vi "XML_FF_writeClassList.vi"(8 "error in (no error)":errorcluster, 10 "ClassList":string[](array[string]), 11 "DOM document in":refnum<k20>) -> (0 "error out":errorcluster, 3 "DOM document out":refnum<k20>)   [LabVIEW 2016, in "XML_EEG_Features.lvlib"]
uses:
  XML_EEG_Features.lvlib
  <vilib>/xml/NI_XML.lvlib
  <resource>/objmgr/DOMUserDefRef.rc
panel:
  # "This VI is a part of BCI Design library, http://www.ru-bci.org \nCopyright © 2020, Sotnikov Peter, All rights reserved. License: CC BY-NC 4.0"
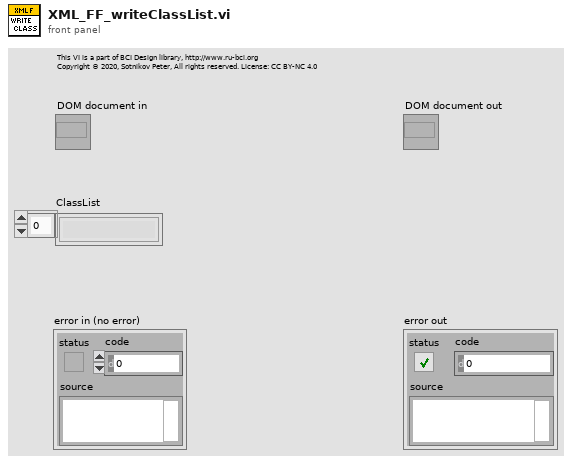
[diagram p1: front panel]
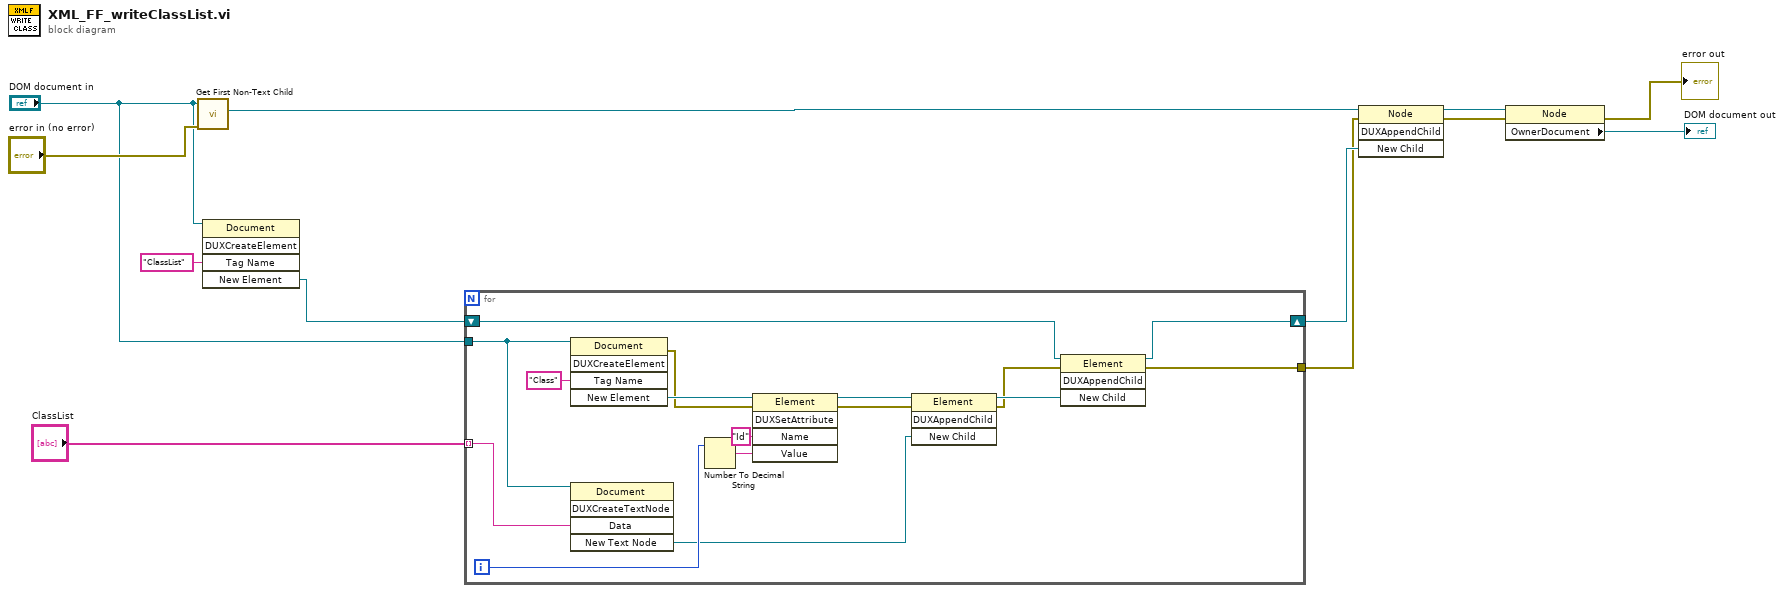
[diagram p0: block diagram]
diagram:
  n1 = call <vilib>:"Get First Non-Text Child.vi"("error in (no error)"="error in (no error)", "node in"="DOM document in") -> ("child node"=w6:refnum<k20>)  [unwired: 6 in, 3 out]
  n2 = invoke class="Document" method="DUXCreateElement"(reference="DOM document in", "Tag Name"="ClassList") -> ("New Element"=w8:refnum<k20>)  [unwired: 3 in, 4 out]
  n3 = for {
    tunnel: "ClassList" -> [w26] mode=indexing
    tunnel: "DOM document in" -> [w27]
    shift-right: [w16] -> w7
    shift-left: w8 -> [w17]
    tunnel: [w13] -> w3
    i -> [w23]
    n4 = invoke class="Document" method="DUXCreateElement"(reference=w27, "Tag Name"="Class") -> (error out=w21:errorcluster, "New Element"=w25:refnum<k20>)  [unwired: 3 in, 3 out]
    n5 = invoke class="Document" method="DUXCreateTextNode"(reference=w27, "Data"=w26) -> ("New Text Node"=w19:refnum<k20>)  [unwired: 3 in, 4 out]
    n6 = Number To Decimal String(number=w23) -> (decimal integer string=w24:string)  [unwired: 1 in]
    n7 = invoke class="Element" method="DUXSetAttribute"(reference=w25, error in=w21, "Name"="Id", "Value"=w24) -> (reference out=w20:refnum<k20>, error out=w15:errorcluster)  [unwired: 1 in, 3 out]
    n8 = invoke class="Element" method="DUXAppendChild"(reference=w20, error in=w15, "New Child"=w19) -> (reference out=w18:refnum<k20>, error out=w14:errorcluster)  [unwired: 1 in, 2 out]
    n9 = invoke class="Element" method="DUXAppendChild"(reference=w17, error in=w14, "New Child"=w18) -> (reference out=w16:refnum<k20>, error out=w13:errorcluster)  [unwired: 1 in, 2 out]
  }
  n10 = invoke class="Node" method="DUXAppendChild"(reference=w6, error in=w3, "New Child"=w7) -> (reference out=w5:refnum<k20>, error out=w4:errorcluster)  [unwired: 1 in, 2 out]
  n11 = property class="Node"(reference=w5, error in=w4) -> (error out=→"error out":errorcluster, "OwnerDocument"=→"DOM document out":refnum<k20>)  [unwired: 1 out]
